vi "ArmBegin.vi"(8 "error in (no error)":errorcluster) -> (0 "error out":errorcluster)   [LabVIEW 2023]
doc: "Arm begin\nOpens ArmLift motor\nInputs:\nNone\nOutputs:\nnone"
uses:
  <vilib>/Rock Robotics/WPI/ThirdParty/REV Robotics/REVLib/Typedef/Spark MAX Idle Mode.ctl
  <vilib>/Rock Robotics/WPI/ThirdParty/REV Robotics/REVLib/Typedef/Spark MAX Limit Switch Polarity.ctl
  <vilib>/Rock Robotics/WPI/Switch/WPI_SwitchOpenLimit.vi
  <vilib>/Rock Robotics/SystemInterfaces/DIO/FPGA_DIOChannel.ctl
  <vilib>/Rock Robotics/WPI/ThirdParty/REV Robotics/REVLib/SubVI/Public/SPARK Configure Basic Ramp Rate.vi
  <vilib>/Rock Robotics/WPI/ThirdParty/REV Robotics/REVLib/SubVI/Public/SPARK Configure Limit Switch Reverse.vi
  <vilib>/Rock Robotics/WPI/ThirdParty/REV Robotics/REVLib/SubVI/Public/SPARK Configure Limit Switch Forward.vi
  <vilib>/Rock Robotics/WPI/ThirdParty/REV Robotics/REVLib/SubVI/Public/SPARK Configure Basic Idle Mode.vi
  <vilib>/Rock Robotics/WPI/ThirdParty/REV Robotics/REVLib/SubVI/Public/SPARK Open Brushless.vi
  <vilib>/Rock Robotics/WPI/ThirdParty/REV Robotics/REVLib/SubVI/Public/SPARK Configure Encoder Conversion Factors.vi
  <vilib>/Rock Robotics/WPI/ThirdParty/REV Robotics/REVLib/SubVI/Public/SPARK Configure Power Smart Current Limit.vi
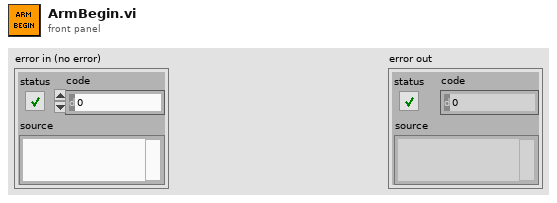
[diagram p1: front panel]
types:
  T1 = typedef "Spark MAX Limit Switch Polarity.ctl" = enum16{"Normally Open", "Normally Closed"}
  T2 = typedef "Spark MAX Idle Mode.ctl" = enum16{"Coast", "Brake"}
  T3 = typedef "FPGA_DIOChannel.ctl" = enum8{"DIO 0", "DIO 1", "DIO 2", "DIO 3", "DIO 4", "DIO 5", "DIO 6", "DIO 7", "DIO 8", "DIO 9", "DIO MXP 0", "DIO MXP 1", "DIO MXP 2", "DIO MXP 3", "DIO MXP 4", "DIO MXP 5", "DIO MXP 6", "DIO MXP 7", "DIO MXP 8", "DIO MXP 9", "DIO MXP 10", "DIO MXP 11", "DIO MXP 12", "DIO MXP 13", "DIO MXP 14", "DIO MXP 15", "SPI Port CS1", "SPI Port CS2", "SPI Port CS3", "SPI Port MISO", "SPI Port MOSI", "Invalid"}
  T4 = typedef "WPI_MotorControlDeviceRef.ctl" = cluster{"DeviceStatus":errorcluster, "Type":T5, "PWM":cluster{"PWM Channel":T6, "DeadBand":T7}, "CAN":cluster{"Device Number":u8, "SetOutput VI Ref":variant, "GetOutput VI Ref":variant, "Enable VI Ref":variant, "Disable VI Ref":variant, "Data":variant}, "Invert":bool, "DIO PWM":cluster{"PWM \"Enable\" Channel":T6, "DIOChannel":T3, "PWM Rate":dbl}}
  T5 = typedef "WPI_MotorControlType.ctl" = enum16{"PWM", "CAN", "DIO PWM"}
  T6 = typedef "FPGA_DIOPWMChannel.ctl" = enum8{"PWM 0", "PWM 1", "PWM 2", "PWM 3", "PWM 4", "PWM 5", "PWM 6", "PWM 7", "PWM 8", "PWM 9", "PWM MXP 0", "PWM MXP 1", "PWM MXP 2", "PWM MXP 3", "PWM MXP 4", "PWM MXP 5", "PWM MXP 6", "PWM MXP 7", "PWM MXP 8", "PWM MXP 9", "Invalid"}
  T7 = typedef "WPI_PWMDeadband.ctl" = cluster{"Name":string, "maxPositivePwm":i32, "minPositivePwm":i32, "centerPwm":i32, "maxNegativePwm":i32, "minNegativePwm":i32, "angularRange":u16}
  T8 = typedef "WPI_SwitchDevRef.ctl" = cluster{"DevStatus":errorcluster, "DIO Channel":T3, "CntIndex":T9, "Normally Closed":bool}
  T9 = typedef "FPGA_CounterCtrSystemIndex.ctl" = enum8{"Ctr 0", "Ctr 1", "Ctr 2", "Ctr 3", "Ctr 4", "Ctr 5", "Ctr 6", "Ctr 7", "Invalid"}
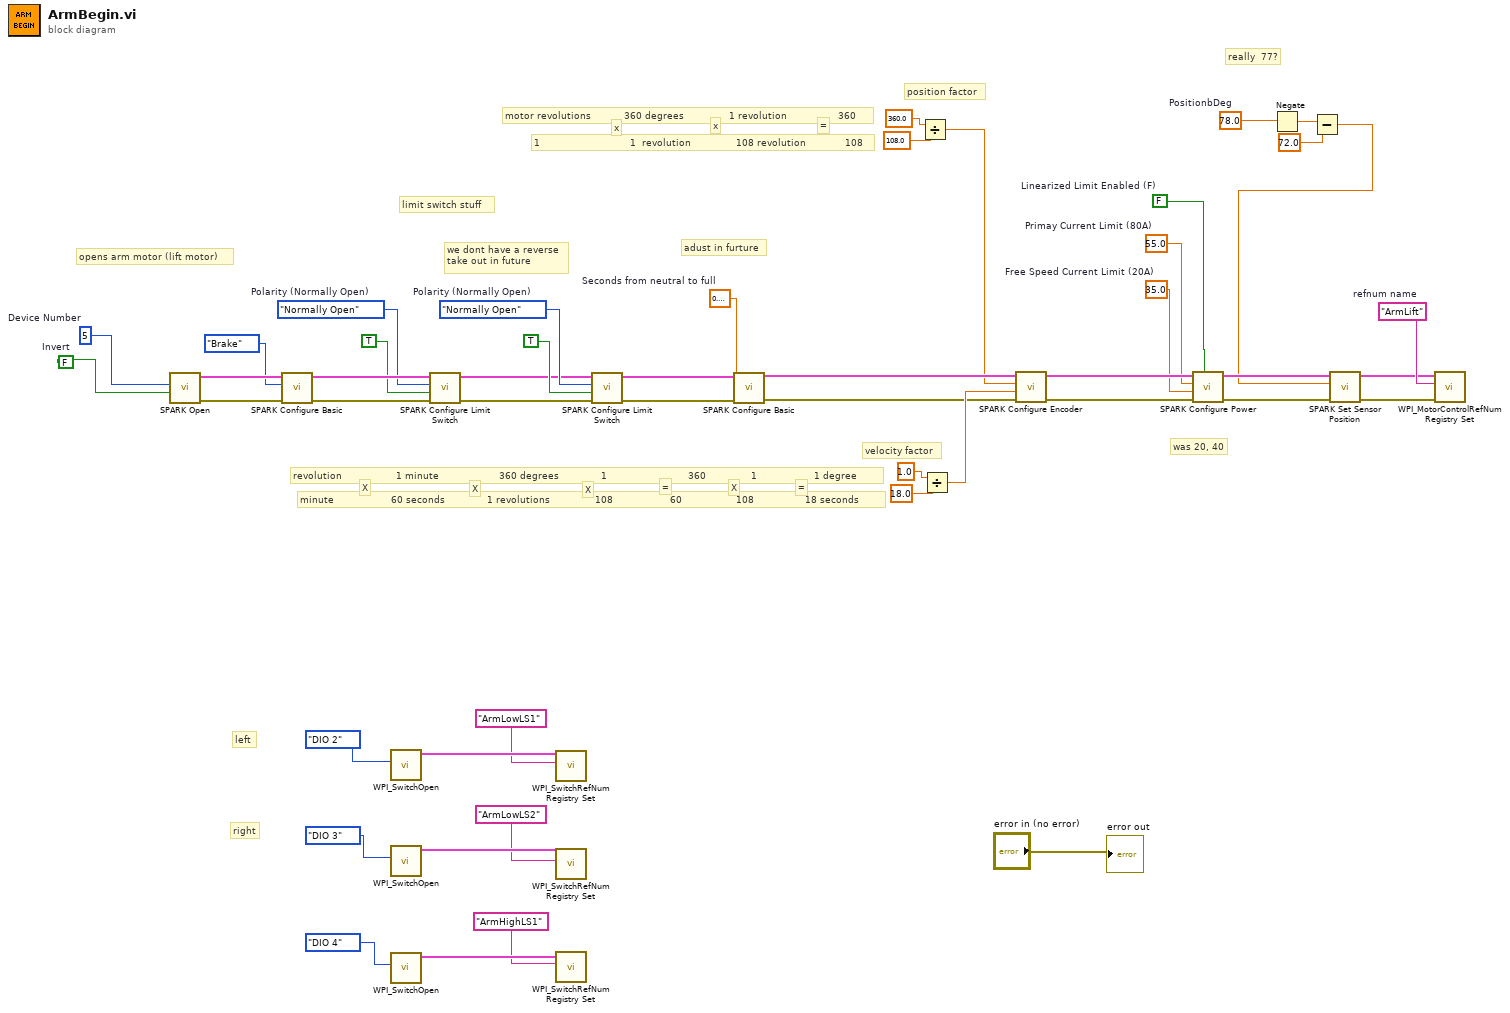
[diagram p0: block diagram]
diagram:
  w17 = Spark_MAX_Limit_Switch_Polarity."Normally Open"  # Polarity (Normally Open)
  w23 = Spark_MAX_Limit_Switch_Polarity."Normally Open"  # Polarity (Normally Open)
  w4 = FALSE  # Linearized Limit Enabled (F)
  w11 = sgl 0.2  # Seconds from neutral to full
  w42 = 78.0  # PositionbDeg
  w48 = "ArmLift"  # refnum name
  w6 = 35.0  # Free Speed Current Limit (20A)
  w5 = 55.0  # Primay Current Limit (80A)
  w18 = FALSE  # Invert
  w19 = u8 5  # Device Number
  # "right"
  # "left"
  # "was 20, 40"
  # "we dont have a reverse\ntake out in future"
  # "adust in furture"
  # "velocity factor"
  # "position factor"
  # "limit switch stuff"
  # "X"
  # "X"
  # "X"
  # "X"
  # "="
  # "="
  # "minute                   60 seconds              1 revolutions               108                   60                  108                 18 seconds"
  # "revolution                  1 minute                    360 degrees              1                           360               1                   1 degree"
  # "1                              1  revolution               108 revolution             108"
  # "="
  # "x"
  # "x"
  # "motor revolutions           360 degrees               1 revolution                 360"
  # "really  77?"
  # "opens arm motor (lift motor)"
  n1 = call-poly <vilib>:"SPARK Open.vi"("Invert"=w18, "Device Number"=w19) -> ("error out"=w29:errorcluster, "MotorControlDeviceRef"=w30:T4)  [unwired: 8 in]
  n2 = call-poly <vilib>:"SPARK Configure Basic.vi"("error in (no error)"=w29, "Idle Mode"=Spark_MAX_Idle_Mode."Brake", "MotorControlDeviceRef in"=w30) -> ("error out"=w24:errorcluster, "MotorControlDeviceRef out"=w25:T4)  [unwired: 7 in]
  n3 = call-poly <vilib>:"WPI_SwitchOpen.vi"("DIO Channel"=FPGA_DIOChannel."DIO 2") -> ("SwitchDevRef"=w39:T8)  [unwired: 9 in, 1 out]
  n4 = call-poly <vilib>:"WPI_SwitchOpen.vi"("DIO Channel"=FPGA_DIOChannel."DIO 3") -> ("SwitchDevRef"=w33:T8)  [unwired: 9 in, 1 out]
  n5 = call-poly <vilib>:"WPI_SwitchOpen.vi"("DIO Channel"=FPGA_DIOChannel."DIO 4") -> ("SwitchDevRef"=w36:T8)  [unwired: 9 in, 1 out]
  n6 = call-poly <vilib>:"SPARK Configure Limit Switch.vi"("error in"=w24, "Enabled? (T)"=TRUE, "Polarity (Normally Open)"=w23, "MotorControlDeviceRef in"=w25) -> ("error out"=w14:errorcluster, "MotorControlDeviceRef out"=w15:T4)  [unwired: 6 in]
  n7 = call <vilib>:"WPI_SwitchRefNum Registry Set.vi"("refnum name"="ArmLowLS1", "SwitchDevRef"=w39) -> ()  [unwired: 8 in, 2 out]
  n8 = call <vilib>:"WPI_SwitchRefNum Registry Set.vi"("refnum name"="ArmLowLS2", "SwitchDevRef"=w33) -> ()  [unwired: 8 in, 2 out]
  n9 = call <vilib>:"WPI_SwitchRefNum Registry Set.vi"("refnum name"="ArmHighLS1", "SwitchDevRef"=w36) -> ()  [unwired: 8 in, 2 out]
  n10 = call-poly <vilib>:"SPARK Configure Limit Switch.vi"("error in"=w14, "Enabled? (T)"=TRUE, "Polarity (Normally Open)"=w17, "MotorControlDeviceRef in"=w15) -> ("error out"=w12:errorcluster, "MotorControlDeviceRef out"=w13:T4)  [unwired: 6 in]
  n11 = call-poly <vilib>:"SPARK Configure Basic.vi"("error in (no error)"=w12, "Seconds from neutral to full (0)"=w11, "MotorControlDeviceRef in"=w13) -> ("error out"=w8:errorcluster, "MotorControlDeviceRef"=w9:T4)  [unwired: 7 in]
  n12 = Divide(x=360.0 ("Velocity Factor (1)"), y=108.0) -> (x/y=w7:dbl)
  n13 = Divide(x=1.0 ("Velocity Factor (1)"), y=18.0) -> (x/y=w10:dbl)
  n14 = call-poly <vilib>:"SPARK Configure Encoder.vi"("error in"=w8, "Velocity Conversion Factor"=w10, "Position Conversion Factor"=w7, "MotorControlDeviceRef in"=w9) -> ("error out"=w26:errorcluster, "MotorControlDeviceRef out"=w27:T4)  [unwired: 6 in]
  n15 = call-poly <vilib>:"SPARK Configure Power.vi"("Linearized Limit Enabled (F)"=w4, "error in (no error)"=w26, "Free Speed Current Limit (20A)"=w6, "Primay Current Limit (80A)"=w5, "MotorControlDeviceRef in"=w27) -> ("error out"=w20:errorcluster, "MotorControlDeviceRef out"=w21:T4)  [unwired: 5 in]
  n16 = Negate(x=w42) -> (-x=w41:dbl)
  n17 = Subtract(x=w41, y=72.0) -> (x-y=w3:dbl)
  n18 = call <vilib>:"SPARK Set Sensor Position.vi"("error in"=w20, "Position"=w3, "MotorControlDeviceRef"=w21) -> ("error out"=w1:errorcluster, "MotorControlDeviceRef"=w2:T4)  [unwired: 7 in]
  n19 = call <vilib>:"WPI_MotorControlRefNum Registry Set.vi"("error in (no error)"=w1, "refnum name"=w48, "MotorControlDevRef"=w2) -> ()  [unwired: 7 in, 2 out]
  "error out" <- "error in (no error)"
